vi "RetaInimigoBola.vi"(1 "DistInFrontGoal":dbl=90.0 format="%#_13g", 4 "Y quina":dbl format="%#_13g", 5 "Meio?":bool=TRUE, 6 "Goal width":u32, 7 "Field lenght":u32, 8 "Y bola":dbl format="%#_13g", 9 "X bola":dbl format="%#_13g", 10 "Y inimigo":dbl format="%#_13g", 11 "X inimigo":dbl format="%#_13g") -> (0 "Orientação":dbl format="%#_13g", 2 "Y goleiro":dbl format="%#_13g", 3 "X goleiro":dbl format="%#_13g")   [LabVIEW 2020]
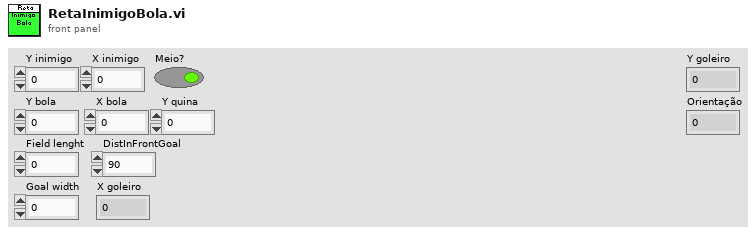
[diagram p1: front panel]
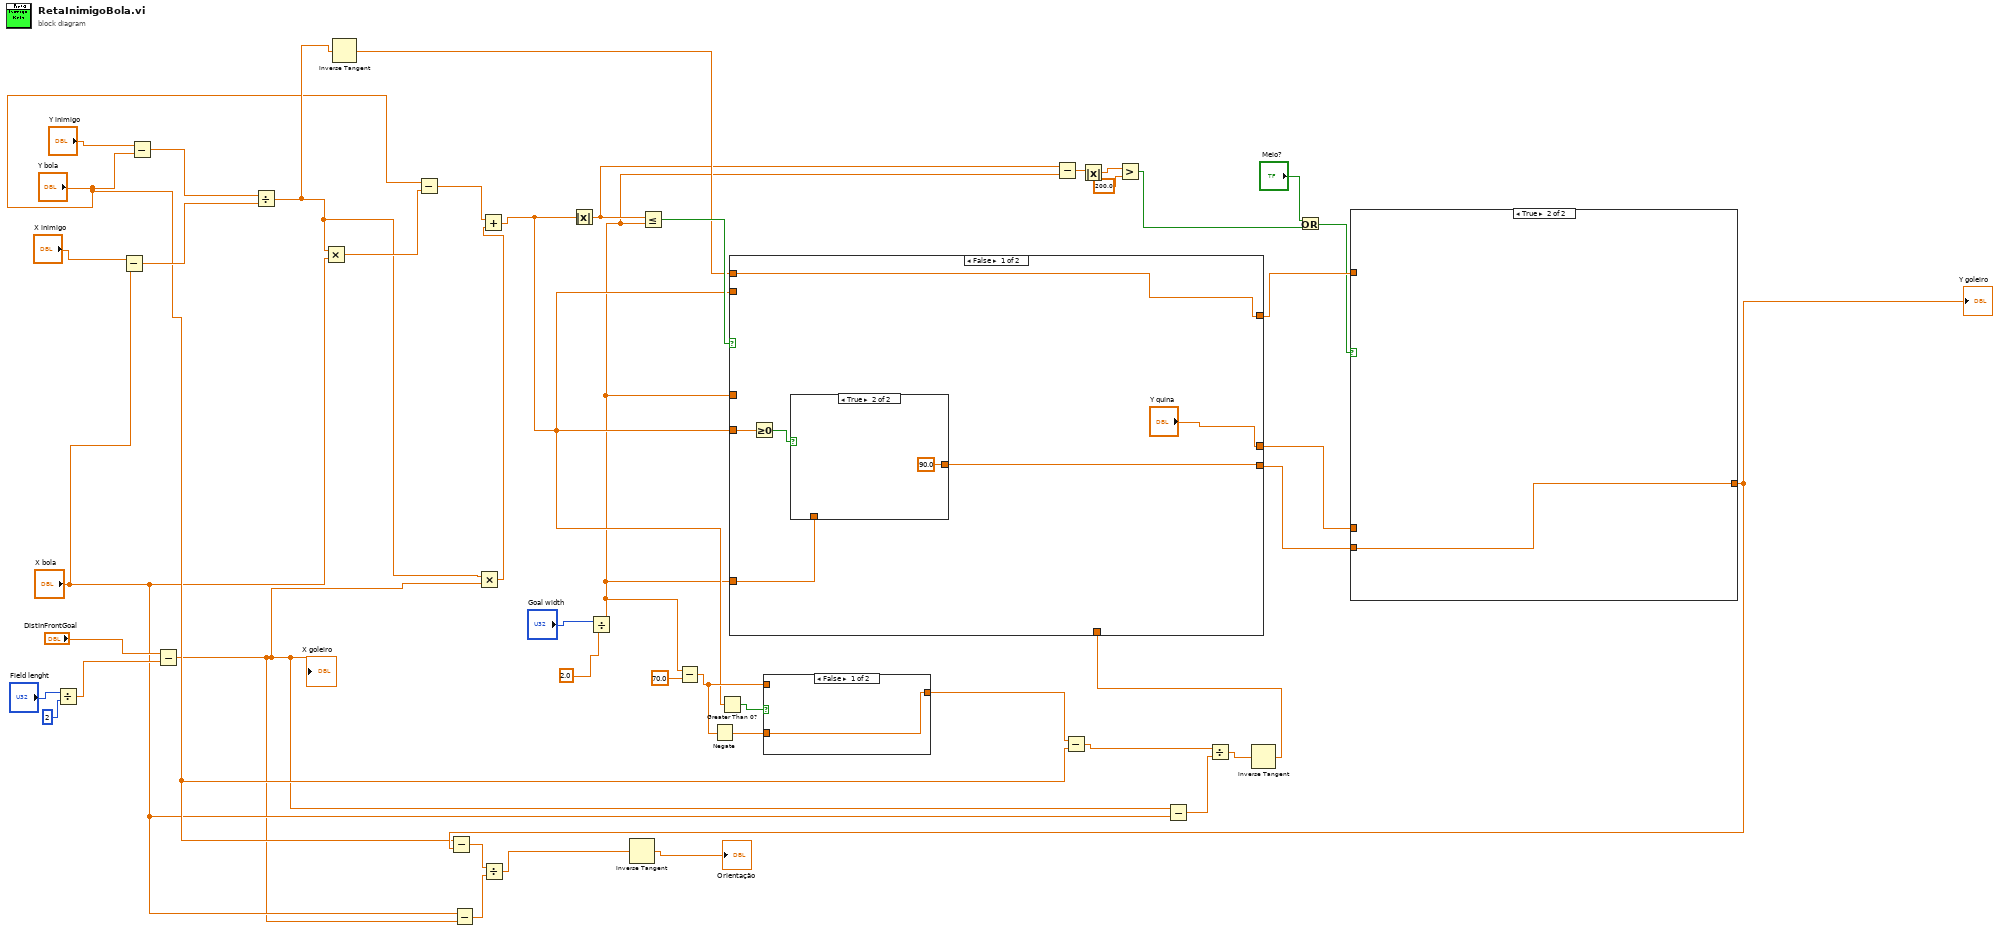
[diagram p0: block diagram]
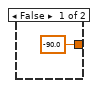
[diagram p4: hidden frame]
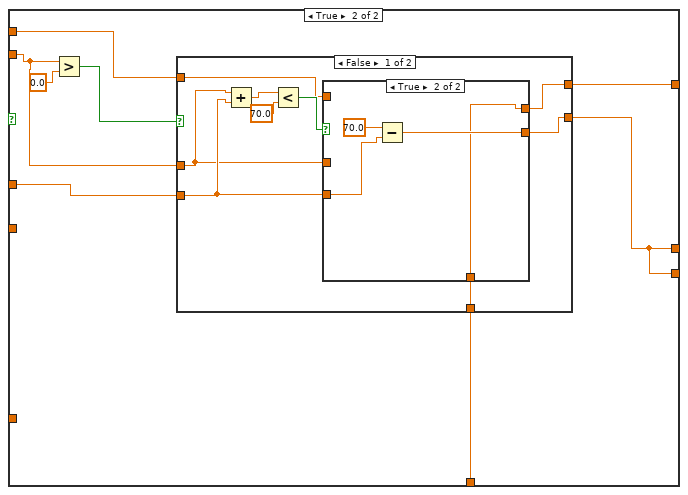
[diagram p5: hidden frame]
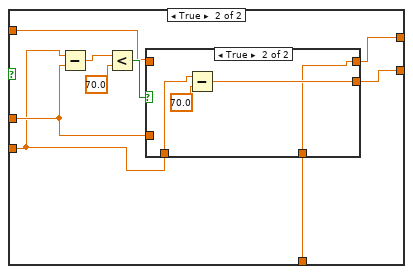
[diagram p7: hidden frame]
diagram:
  n1 = Divide(x="Field lenght", y=2) -> (x/y=w37:dbl)
  n2 = Subtract(x="X inimigo", y="X bola") -> (x-y=w42:dbl)
  n3 = Subtract(x="Y inimigo", y="Y bola") -> (x-y=w43:dbl)
  n4 = Subtract(x="DistInFrontGoal", y=w37) -> (x-y=w9:dbl)
  "X goleiro" <- w9
  n5 = Divide(x=w43, y=w42) -> (x/y=w31:dbl)
  n6 = Multiply(x=w31, y="X bola") -> (x*y=w41:dbl)
  n7 = Inverse Tangent(1:w31) -> (0:w30:dbl)
  n8 = Subtract(x="Y bola", y=w41) -> (x-y=w36:dbl)
  n9 = Subtract(x="X bola", y=w9) -> (x-y=w11:dbl)
  n10 = Multiply(x=w31, y=w9) -> (x*y=w35:dbl)
  n11 = Add(x=w36, y=w35) -> (x+y=w17:dbl)
  n12 = Absolute Value(x=w17) -> (abs(x)=w5:dbl)
  n13 = Divide(x="Goal width", y=2.0) -> (x/y=w4:dbl)
  n14 = Less Or Equal?(x=w5, y=w4) -> (x <= y?=w34:bool)
  n15 = Subtract(x=w4, y=70.0) -> (x-y=w26:dbl)
  n16 = Negate(x=w26) -> (-x=w25:dbl)
  n17 = Greater Than 0?(x=w17) -> (x > 0?=w28:bool)
  n18 = case shown="False" w28 {
    tunnel: w26 -> [_ w47]
    tunnel: [w46 w47] -> w27
    tunnel: w25 -> [w46 _]
    frame False {
    }
    frame True {
    }
  }
  n19 = Subtract(x=w5, y=w4) -> (x-y=w8:dbl)
  n20 = Subtract(x=w27, y="Y bola") -> (x-y=w24:dbl)
  n21 = Absolute Value(x=w8) -> (abs(x)=w7:dbl)
  n22 = Greater?(x=w7, y=200.0) -> (0:w2:bool)
  n23 = Subtract(x=w9, y="X bola") -> (x-y=w23:dbl)
  n24 = Divide(x=w24, y=w23) -> (x/y=w22:dbl)
  n25 = Inverse Tangent(1:w22) -> (0:w21:dbl)
  n26 = case shown="False" w34 {
    tunnel: ["Y quina" w56] -> w19
    tunnel: w17 -> [_ w60]
    tunnel: w4 -> [_ w61]
    tunnel: w30 -> [w53 w59]
    tunnel: [w53 w58] -> w20
    tunnel: w21 -> [_ w57]
    tunnel: [w49 w56] -> w18
    tunnel: w17 -> [w52 _]
    tunnel: w4 -> [w50 _]
    frame False {
      n27 = Greater Or Equal To 0?(x=w52) -> (x >= 0?=w51:bool)
      n28 = case shown="True" w51 {
        tunnel: w50 -> [_ _]
        tunnel: [-90.0 90.0] -> w49
        frame False {
        }
        frame True {
        }
      }
    }
    frame True {
      n29 = Greater?(x=w60, y=0.0) -> (0:w62:bool)
      n30 = case shown="False" w62 {
        tunnel: w61 -> [w69 w82]
        tunnel: w60 -> [w67 w83]
        tunnel: [w68 w84] -> w56
        tunnel: w59 -> [w66 w81]
        tunnel: [w65 w80] -> w58
        tunnel: w57 -> [w64 w79]
        frame False {
          n31 = Add(x=w67, y=w69) -> (x+y=w72:dbl)
          n32 = Less?(x=w72, y=70.0) -> (x < y?=w70:bool)
          n33 = case shown="True" w70 {
            tunnel: w69 -> [_ w77]
            tunnel: [w74 w76] -> w68
            tunnel: w67 -> [w74 _]
            tunnel: w66 -> [w73 _]
            tunnel: [w73 w75] -> w65
            tunnel: w64 -> [_ w75]
            frame False {
            }
            frame True {
              n34 = Subtract(x=70.0, y=w77) -> (x-y=w76:dbl)
            }
          }
        }
        frame True {
          n35 = Subtract(x=w82, y=w83) -> (x-y=w87:dbl)
          n36 = Less?(x=w87, y=70.0) -> (x < y?=w85:bool)
          n37 = case shown="True" w85 {
            tunnel: [w89 w92] -> w84
            tunnel: w83 -> [w89 _]
            tunnel: w82 -> [_ w91]
            tunnel: w81 -> [w88 _]
            tunnel: [w88 w90] -> w80
            tunnel: w79 -> [_ w90]
            frame False {
            }
            frame True {
              n38 = Subtract(x=w91, y=70.0) -> (x-y=w92:dbl)
            }
          }
        }
      }
    }
  }
  n39 = Or(x="Meio?", y=w2) -> (x .or. y?=w1:bool)
  n40 = case shown="True" w1 {
    tunnel: w20 -> [_ _]
    tunnel: [w94 w95] -> w15
    tunnel: w19 -> [w94 _]
    tunnel: w18 -> [_ w95]
    frame False {
    }
    frame True {
    }
  }
  "Y goleiro" <- w15
  n41 = Subtract(x="Y bola", y=w15) -> (x-y=w12:dbl)
  n42 = Divide(x=w12, y=w11) -> (x/y=w10:dbl)
  n43 = Inverse Tangent(1:w10) -> (0:→"Orientação":dbl)
